vi "get_max_-max2.vi"(3 "Waveform out":T1) -> (0 "-max_xy":dbl, 1 "max_xy":dbl)   [LabVIEW 2013]
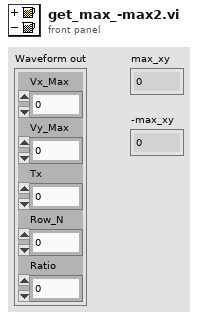
[diagram p1: front panel]
types:
  T1 = cluster{"Vx_Max":dbl, "Vy_Max":dbl, "Tx":dbl, "Row_N":i32, "Ratio":dbl}
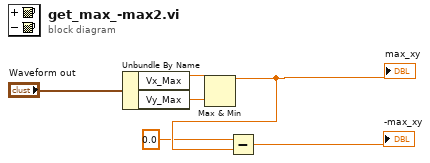
[diagram p0: block diagram]
diagram:
  n1 = Unbundle By Name("Waveform out") -> ("Vx_Max"=w3:dbl, "Vy_Max"=w4:dbl)
  n2 = Max & Min(x=w3, y=w4) -> (max(x,y)=w5:dbl)  [unwired: 1 out]
  "max_xy" <- w5
  n3 = Subtract(x=0.0, y=w5) -> (x-y=→"-max_xy":dbl)
